vi "Test Harness.vi"() -> ()   [LabVIEW 2015, in "Generic Module Library.lvlib" / "Template G_Module.lvlib"]
uses:
  Template G_Module.lvlib
panel:
  out "Closing Response":string
  out "Response":string
  out "Timed Out":bool
  out "Sending Timestamp":timestamp
  out "Broadcast Timestamp":timestamp
  in  "Ping Module":bool
  in  "Stop Module":bool
  # "Test API Calls"
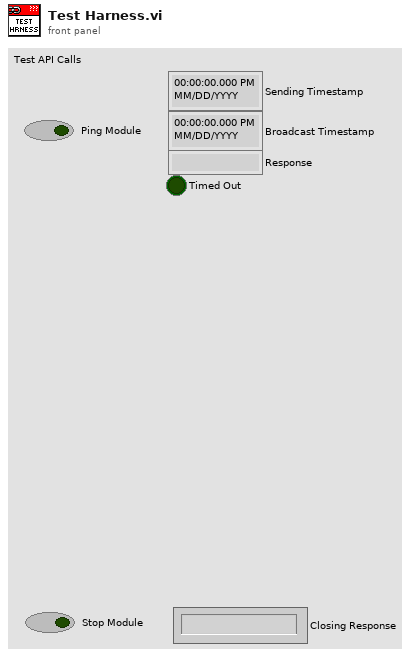
[diagram p1: front panel]
types:
  T1 = typedef "Generic Module Library.lvlib/Template G_Module.lvlib/Broadcast List.ctl" = cluster{"Module Started":refnum<user-event>, "Module Error":refnum<user-event>, "Module Pong":refnum<user-event>, "Module Status":refnum<user-event>, "Module Stopping":refnum<user-event>, "Module Stopped":refnum<user-event>, "Module Reinitialized":refnum<user-event>}
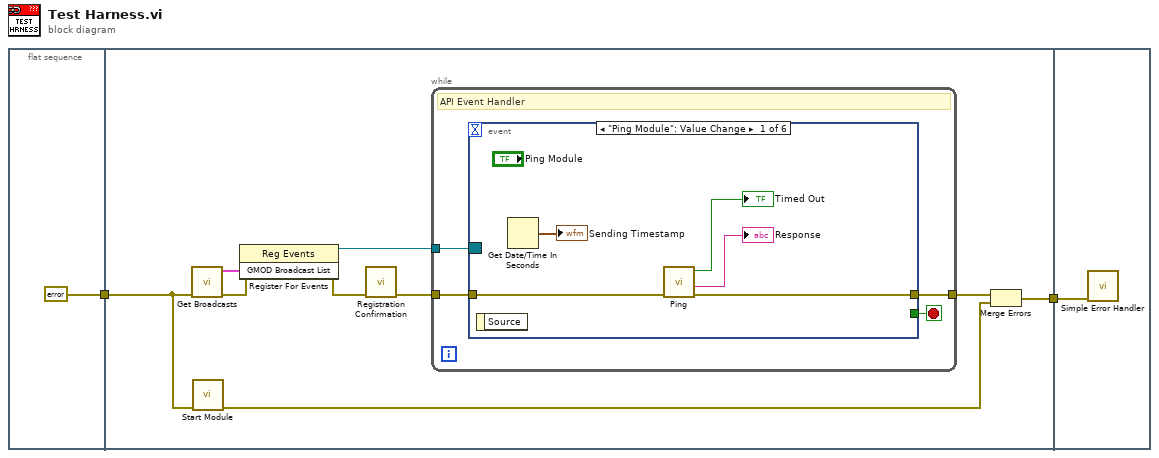
[diagram p0: block diagram]
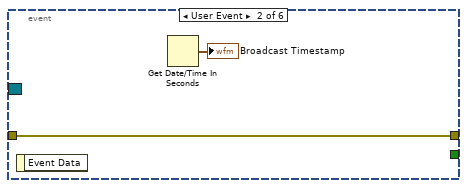
[diagram p2: hidden frame]
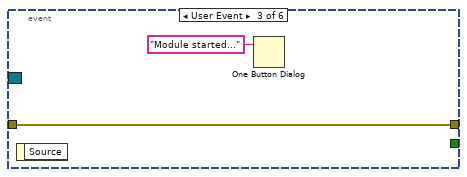
[diagram p3: hidden frame]
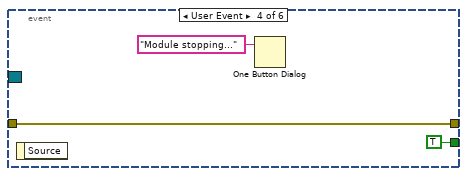
[diagram p4: hidden frame]
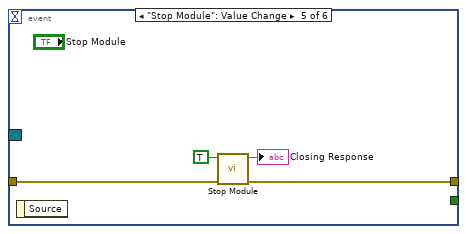
[diagram p5: hidden frame]
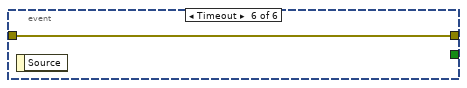
[diagram p6: hidden frame]
diagram:
  n1 = flat-sequence {
    tunnel: [errorcluster {"status"=FALSE, "code"=0, "source"=""} ("error in (no error)")] -> w1
    tunnel: [w10] -> w2
    tunnel: w1 -> [w6]
    tunnel: w2 -> [w34]
    frame #0 {
    }
    frame #1 {
      n2 = call "Get Broadcasts.vi"("error in (no error)"=w6) -> ("error out"=w9:errorcluster, "GMOD Broadcast List"=w8:T1)  [unwired: 8 in, 1 out]
      n3 = call "Start Module.vi"("error in (no error)"=w6) -> ("error out"=w11:errorcluster)  [unwired: 9 in, 1 out]
      n4 = register-events(error in=w9, w8) -> (reference out=w7:refnum<event-registration>, error out=w5:errorcluster)  [unwired: 1 in]
      n5 = call "Registration Confirmation.vi"("error in"=w5) -> ("error out"=w4:errorcluster)  [unwired: 10 in]
      n6 = while {
        tunnel: w7 -> [w13]
        tunnel: w4 -> [w15]
        tunnel: [w14] -> w12
        stop <- w16 stop-if-true
        # "API Event Handler"
        n7 = event shown="[0] \"Ping Module\": Value Change" {
          selector: w13 -> [_ _ _ _ _ _]
          dyn-events: _ -> [_ _ _ _ _ _]
          timeout: _ -> [_ _ _ _ _ _]
          tunnel: [_ _ _ TRUE _ _] -> w16
          tunnel: w15 -> [w21 w23 w25 w28 w32 w33]
          tunnel: [w18 w23 w25 w28 w31 w33] -> w14
          event "Ping Module": Value Change {
            n8 = event-data() -> ()  [unwired: 1 in, 1 out]
            n9 = Get Date/Time In Seconds() -> (seconds since 1Jan1904=→"Sending Timestamp":timestamp)
            n10 = call "Ping.vi"("error in"=w21) -> ("error out"=w18:errorcluster, "Response"=→"Response":string, "Timed Out"=→"Timed Out":bool)  [unwired: 8 in]
          }
          event User Event {
            n11 = event-data() -> ()  [unwired: 1 in, 1 out]
            n12 = Get Date/Time In Seconds() -> (seconds since 1Jan1904=→"Broadcast Timestamp":timestamp)
          }
          event User Event {
            n13 = event-data() -> ()  [unwired: 1 in, 1 out]
            n14 = One Button Dialog(message="Module started...") -> ()  [unwired: 1 in, 1 out]
          }
          event User Event {
            n15 = event-data() -> ()  [unwired: 1 in, 1 out]
            n16 = One Button Dialog(message="Module stopping...") -> ()  [unwired: 1 in, 1 out]
          }
          event "Stop Module": Value Change {
            n17 = event-data() -> ()  [unwired: 1 in, 1 out]
            n18 = call "Stop Module.vi"("error in (no error)"=w32, "Wait for Stop Execution?"=TRUE) -> ("error out"=w31:errorcluster, "Response"=→"Closing Response":string)  [unwired: 8 in]
          }
          event Timeout {
            n19 = event-data() -> ()  [unwired: 1 in, 1 out]
          }
        }
      }
      n20 = Merge Errors(w12, w11) -> (w10:errorcluster)
    }
    frame #2 {
      n21 = call <vilib>:"Simple Error Handler.vi"("error in (no error)"=w34) -> ()  [unwired: 4 in, 5 out]
    }
  }
